vi "MGI SZL Add File.vi"(4 "compressionMethod (Deflated)":i32(ring)=8 items=["Stored"=0, "Deflated"=8, "Deflate64"=9, "BZip2"=11, "WinZipAES"=99], 6 "updateMode (Safe)":i32(ring) items=["Safe", "Direct"], 8 "Error In":errorcluster, 9 "Destination Path In Zip":path, 10 "Source File Path":path, 11 "Zip File In":refnum<k24>) -> (0 "Error Out":errorcluster, 3 "Zip File Out":refnum<k24>)   [LabVIEW 2016]
doc: "Adds the file specified by source file path to the zip file. Destination path in zip should be the relative path in the zip file including the name of the file itself, but not including the name of the zip file.\n\nThe updateMode input selects between Safe and Direct. Safe mode will create a temporary file so that errors in the add will not corrupt the entire file. Direct simply adds to the file, so it is more dangerous, but can be significantly faster, particularly for large files.\n\nThis VI relies on the Sharp Zip Library which is a .NET assembly written in C# by Mike Krueger. It is licenced under the GPL with a special exception permitting independent modules to link to the library regardless of the license terms of the independent module. \n\nMore information about the library and its license is available from:\nhttp://www.icsharpcode.net/opensource/sharpziplib/\n\nAuthored by Matthew G. Harrison\nsupport@mooregoodideas.com\nwww.mooregoodideas.com\n\nCopyright (c) 2010, Moore Good Ideas, Inc.\n\nAll rights reserved.\n\nRedistribution and use in source and binary forms, with or without modification, are permitted provided that the following conditions are met:\n\n * Redistributions of source code must retain the above copyright notice, this list of conditions and the following disclaimer.\n * Redistributions in binary form must reproduce the above copyright notice, this list of conditions and the following disclaimer in the documentation and/or other materials provided with the distribution.\n * Neither the name of Moore Good Ideas, Inc. nor the names of its contributors may be used to endorse or promote products derived from this software without specific prior written permission.\n\nTHIS SOFTWARE IS PROVIDED BY THE COPYRIGHT HOLDERS AND CONTRIBUTORS \"AS IS\" AND ANY EXPRESS OR IMPLIED WARRANTIES, INCLUDING, BUT NOT LIMITED TO, THE IMPLIED WARRANTIES OF MERCHANTABILITY AND FITNESS FOR A PARTICULAR PURPOSE ARE DISCLAIMED. IN NO EVENT SHALL THE COPYRIGHT OWNER OR CONTRIBUTORS BE LIABLE FOR ANY DIRECT, INDIRECT, INCIDENTAL, SPECIAL, EXEMPLARY, OR CONSEQUENTIAL DAMAGES (INCLUDING, BUT NOT LIMITED TO, PROCUREMENT OF SUBSTITUTE GOODS OR SERVICES; LOSS OF USE, DATA, OR PROFITS; OR BUSINESS INTERRUPTION) HOWEVER CAUSED AND ON ANY THEORY OF LIABILITY, WHETHER IN CONTRACT, STRICT LIABILITY, OR TORT (INCLUDING NEGLIGENCE OR OTHERWISE) ARISING IN ANY WAY OUT OF THE USE OF THIS SOFTWARE, EVEN IF ADVISED OF THE POSSIBILITY OF SUCH DAMAGE."
uses:
  C:/Program Files (x86)/National Instruments/LabVIEW 2016/user.lib/_MGI/File/Zip/Support Files/ICSharpCode.SharpZipLib.dll
  Support Files/ICSharpCode.SharpZipLib.dll
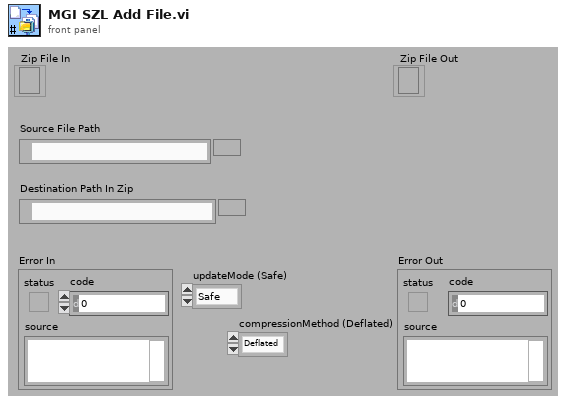
[diagram p1: front panel]
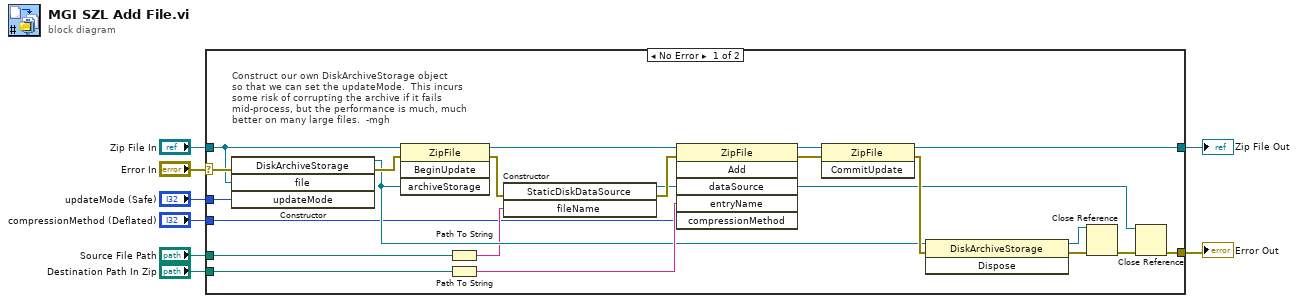
[diagram p0: block diagram]
diagram:
  n1 = case shown="No Error" "Error In" {
    selector: "Error In" -> [w23 w32]
    tunnel: "Zip File In" -> [w18 w31]
    tunnel: "Source File Path" -> [w30 _]
    tunnel: [w11 w32] -> w6
    tunnel: [w25 w31] -> w5
    tunnel: "Destination Path In Zip" -> [w29 _]
    tunnel: "updateMode (Safe)" -> [w19 _]
    tunnel: "compressionMethod (Deflated)" -> [w14 _]
    frame No Error {
      # "Construct our own DiskArchiveStorage object\nso that we can set the updateMode.  This incurs\nsome risk of corrupting the archive if it fails\nmid-process, but the performance is much, much\nbetter on many large files.  -mgh"
      n2 = constructor class="DiskArchiveStorage"(error in=w23, "file"=w18, "updateMode"=w19) -> (reference out=w20:refnum<k24>, error out=w24:errorcluster)  [unwired: 2 in, 3 out]
      n3 = invoke class="ZipFile" method="BeginUpdate"(reference=w18, error in=w24, "archiveStorage"=w20) -> (reference out=w22:refnum<k24>, error out=w16:errorcluster)  [unwired: 1 in, 2 out]
      n4 = Path To String(path=w30) -> (string=w17:string)
      n5 = Path To String(path=w29) -> (string=w28:string)
      n6 = constructor class="StaticDiskDataSource"(error in=w16, "fileName"=w17) -> (reference out=w9:refnum<k24>, error out=w15:errorcluster)  [unwired: 2 in, 2 out]
      n7 = invoke class="ZipFile" method="Add"(reference=w22, error in=w15, "dataSource"=w9, "entryName"=w28, "compressionMethod"=w14) -> (reference out=w27:refnum<k24>, error out=w26:errorcluster)  [unwired: 1 in, 4 out]
      n8 = invoke class="ZipFile" method="CommitUpdate"(reference=w27, error in=w26) -> (reference out=w25:refnum<k24>, error out=w21:errorcluster)  [unwired: 1 in, 1 out]
      n9 = invoke class="DiskArchiveStorage" method="Dispose"(reference=w20, error in=w21) -> (reference out=w12:refnum<k24>, error out=w13:errorcluster)  [unwired: 1 in, 1 out]
      n10 = Close Reference(reference=w12, error in (no error)=w13) -> (error out=w10:errorcluster)
      n11 = Close Reference(reference=w9, error in (no error)=w10) -> (error out=w11:errorcluster)
    }
    frame Error {
    }
  }
  "Error Out" <- w6
  "Zip File Out" <- w5
